vi "Process.vi"(8 "error in (no error)":errorcluster, 10 "pound in":refnum<class "Pound.lvclass">, 11 "qbus in":refnum<class "Qbus.lvclass">) -> (0 "error out":errorcluster)   [LabVIEW 2017, in "SinglePointClock.lvlib"]
doc: "This process sends data sets to the first process in the Dataflow Script for data groups that contain only single-point channels."
uses:
  <vilib>/addons/InsightCM/Devices/Shared/Common/SinglePointClock/SinglePointClock.lvlib
  <vilib>/addons/Qbus/Qbus.lvclass
  <vilib>/NI/Software Watchdog/Pound/Pound.lvclass
  <vilib>/addons/InsightCM/Devices/Shared/Common/SinglePointClock/controls/SinglePointConfig.ctl
  <vilib>/addons/TimerProcess/controls/taskType.ctl
  <vilib>/addons/InsightCM/Devices/Shared/Common/DataFlow/controls/Data.ctl
  <vilib>/addons/InsightCM/Utilities/DataAccessors/controls/wfmSGL_DVR.ctl
  <vilib>/addons/PointValueMap/controls/PointMap.ctl
  <vilib>/addons/InsightCM/Devices/Shared/Common/DataFlow/controls/Type.ctl
  <vilib>/addons/PointValueMap/subVIs/Point_Write_i32.vi
  <vilib>/addons/PointValueMap/subVIs/Point_Write_double.vi
  <vilib>/addons/TraceLogger/TraceLogger.lvlib
  <vilib>/NI/Software Watchdog/Watchdog/Watchdog.lvclass
  <vilib>/addons/InsightCM/Devices/Shared/Common/DataFlow/DataFlow.lvlib
  <vilib>/addons/PointValueMap/PointValueMap.lvlib
  <vilib>/addons/TimerProcess/TimerProcess.lvlib
  <vilib>/addons/InsightCM/Utilities/GlobalConfiguration/GlobalConfiguration.lvlib
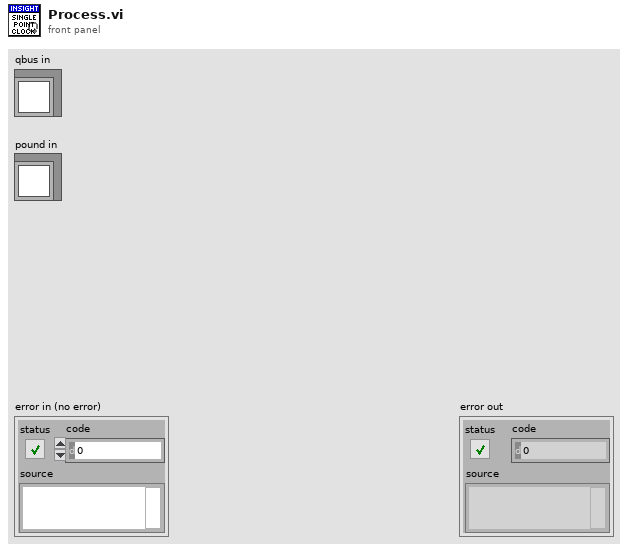
[diagram p1: front panel]
types:
  T1 = typedef "SinglePointConfig.ctl" = cluster{"AcqBlockNumber":i32, "Interval":dbl, "DataGroups":string[], "On":bool}
  T2 = typedef "TimerProcess.lvlib/taskType.ctl" = enum16{"single", "repeat"}
  T3 = typedef "DataFlow.lvlib/Type.ctl" = enum16{"High Rate", "Low Rate", "Burst Mode"}
  T4 = typedef "DataFlow.lvlib/Data.ctl" = cluster{"DataGroup":string, "Waveforms":T5, "Map":T6, "Type":T3}
  T5 = typedef "wfmSGL_DVR.ctl" = refnum<data-value>
  T6 = typedef "PointValueMap.lvlib/PointMap.ctl" = refnum<data-value>
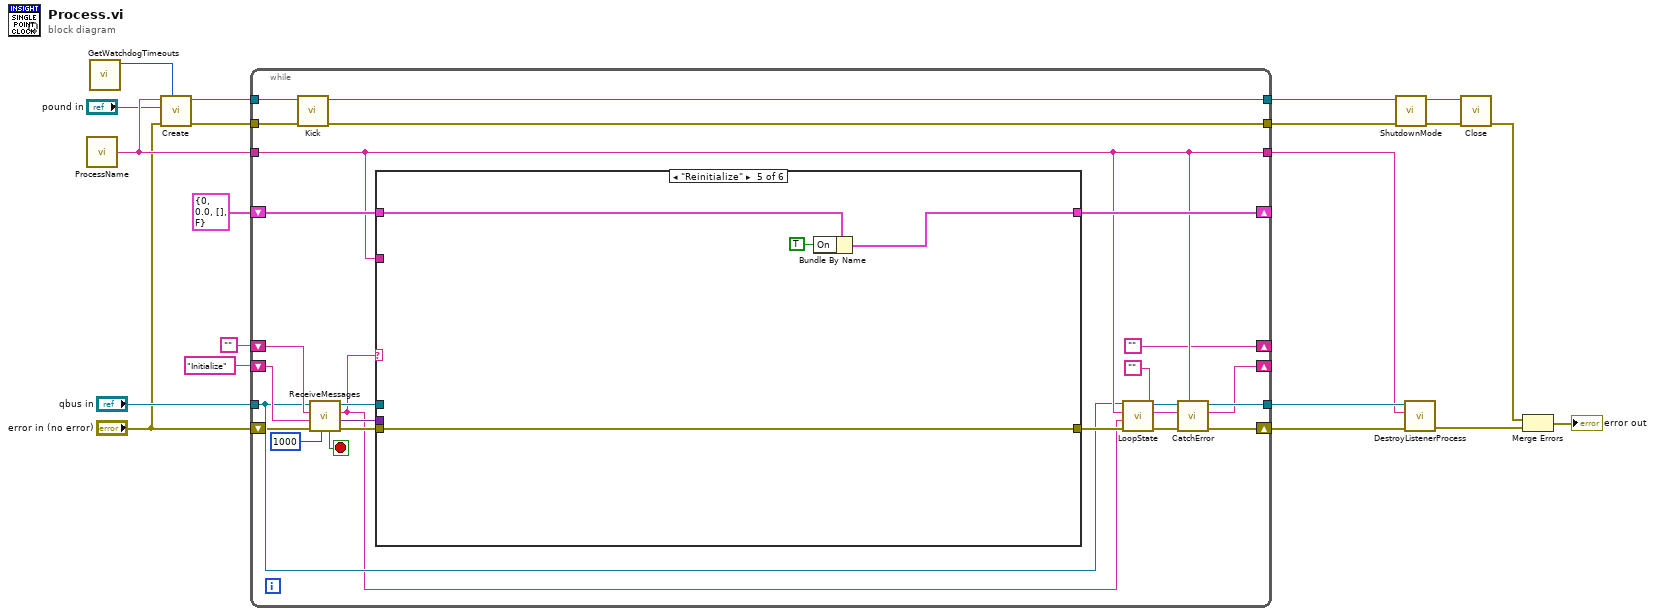
[diagram p0: block diagram]
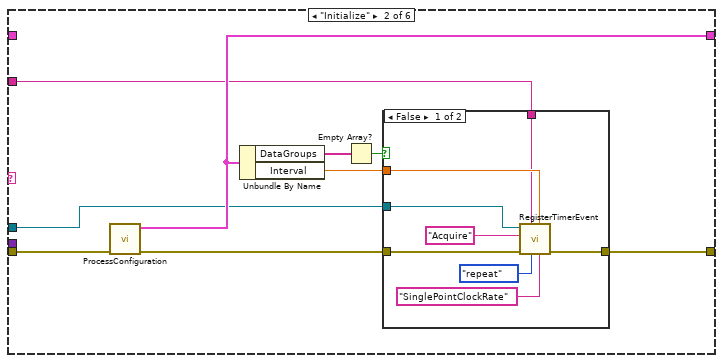
[diagram p3: hidden frame]
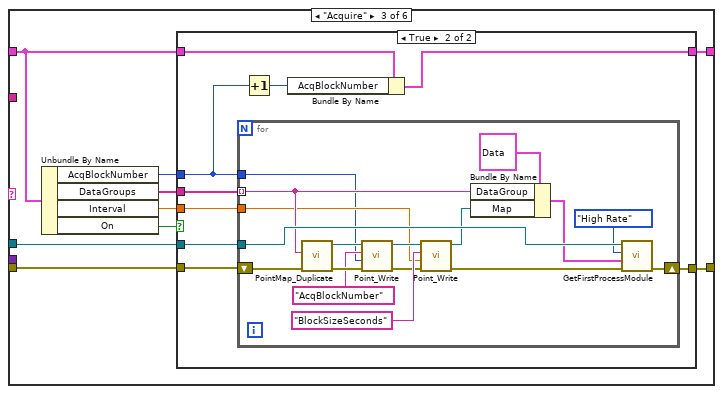
[diagram p5: hidden frame]
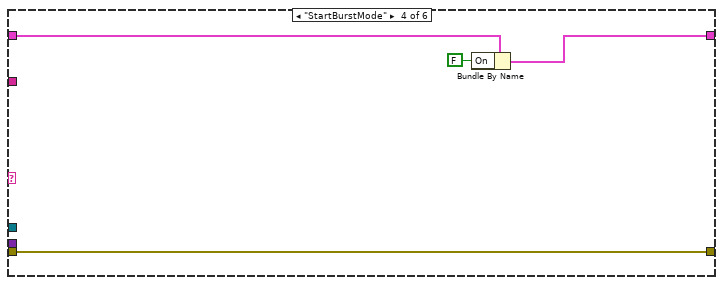
[diagram p7: hidden frame]
diagram:
  n1 = call <vilib>:"ProcessName.vi"() -> ("process name"=w15:string)  [unwired: 5 in]
  n2 = call <vilib>:"GetWatchdogTimeouts.vi"() -> ("software timeout"=w1:u32)  [unwired: 10 in, 1 out]
  n3 = call <vilib>:"Create.vi"("Execution Timeout (ms)"=w1, "error in (no error)"="error in (no error)", "Pound"="pound in", "Name"=w15) -> ("error out"=w9:errorcluster, "Watchdog"=w14:refnum<data-value>)  [unwired: 6 in]
  n4 = while {
    shift-right: [""] -> _
    shift-left: "" -> [w44]
    tunnel: "qbus in" -> [w32]
    tunnel: w15 -> [w33]
    tunnel: [w36] -> w18
    tunnel: [w33] -> w17
    shift-right: [w35] -> _
    shift-left: "Initialize" -> [w40]
    shift-right: [w38] -> _
    shift-left: T1 {"AcqBlockNumber"=0, "Interval"=0.0, "DataGroups"=[], "On"=FALSE} ("Cluster") -> [w39]
    tunnel: w14 -> [w31]
    tunnel: [w30] -> w11
    tunnel: w9 -> [w29]
    tunnel: [w27] -> w8
    shift-right: [w37] -> w19
    shift-left: "error in (no error)" -> [w28]
    stop <- w45 stop-if-true
    n5 = call <vilib>:"Kick.vi"("error in (no error)"=w29, "Watchdog"=w31) -> ("error out"=w27:errorcluster, "Watchdog"=w30:refnum<data-value>)  [unwired: 8 in]
    n6 = call <vilib>:"ReceiveMessages.vi"("timeout(100)"=1000, "error in (no error)"=w28, "priority action"=w40, "default action"=w44, "qbus in"=w32) -> ("error out"=w43:errorcluster, "msg value"=w41:variant, "action"=w26:string, "qbus out"=w42:refnum<class "Qbus.lvclass">, "exit"=w45:bool)  [unwired: 2 in]
    n7 = case shown="\"Reinitialize\"" w26 {
      tunnel: w43 -> [w47 w56 w74 w106 w110 w112]
      tunnel: w42 -> [_ w50 w73 _ _ _]
      tunnel: [w47 w54 w72 w106 w110 w112] -> w34
      tunnel: w41 -> [_ _ _ _ _ _]
      tunnel: w39 -> [w46 _ w70 w105 w109 w111]
      tunnel: [w46 w53 w69 w104 w108 w111] -> w38
      tunnel: w33 -> [_ w51 _ _ _ _]
      frame "", Default {
      }
      frame "Initialize" {
        n8 = call <vilib>:"ProcessConfiguration.vi"("error in (no error)"=w56) -> ("error out"=w55:errorcluster, "config"=w53:T1)  [unwired: 9 in]
        n9 = Unbundle By Name(w53) -> ("DataGroups"=w49:string[], "Interval"=w52:dbl)
        n10 = Empty Array?(array=w49) -> (empty?=w48:bool)
        n11 = case shown="False" w48 {
          tunnel: w55 -> [w61 w65]
          tunnel: [w60 w65] -> w54
          tunnel: w52 -> [w59 _]
          tunnel: w51 -> [w58 _]
          tunnel: w50 -> [w57 _]
          frame False {
            n12 = call <vilib>:"RegisterTimerEvent.vi"("timer task name"="SinglePointClockRate" ("Name"), "interval (sec)"=w59, "type"=taskType."repeat", "process name"=w58, "error in (no error)"=w61, "callback action"="Acquire", "qbus in"=w57) -> ("error out"=w60:errorcluster)  [unwired: 3 in, 1 out]
          }
          frame True {
          }
        }
      }
      frame "Acquire" {
        n13 = Unbundle By Name(w70) -> ("AcqBlockNumber"=w67:i32, "DataGroups"=w71:string[], "Interval"=w68:dbl, "On"=w66:bool)
        n14 = case shown="True" w66 {
          tunnel: w74 -> [w75 w85]
          tunnel: w73 -> [_ w84]
          tunnel: [w75 w83] -> w72
          tunnel: w71 -> [_ w82]
          tunnel: w70 -> [w76 w80]
          tunnel: [w76 w79] -> w69
          tunnel: w68 -> [_ w78]
          tunnel: w67 -> [_ w77]
          frame False {
          }
          frame True {
            n15 = for {
              tunnel: w84 -> [w102]
              shift-right: [w101] -> w83
              shift-left: w85 -> [w96]
              tunnel: w82 -> [w89] mode=indexing
              tunnel: w78 -> [w88]
              tunnel: w77 -> [w87]
              n16 = call <vilib>:"PointMap_Duplicate.vi"("error in (no error)"=w96, "Source Map Name"=w89) -> ("error out"=w91:errorcluster, "Map Out"=w94:T6)  [unwired: 8 in]
              n17 = call-poly <vilib>:"Point_Write.vi"("Error In"=w91, "Value"=w87, "Tag"="AcqBlockNumber", "Map"=w94) -> ("Error Out"=w92:errorcluster, "Map Out"=w93:T6)  [unwired: 6 in]
              n18 = call-poly <vilib>:"Point_Write.vi"("Error In"=w92, "Value"=w88, "Tag"="BlockSizeSeconds", "Map"=w93) -> ("Error Out"=w99:errorcluster, "Map Out"=w98:T6)  [unwired: 6 in]
              n19 = Bundle By Name(cluster=T4 {"DataGroup"="", "Waveforms"=refnum, "Map"=refnum, "Type"=enum."High Rate"} ("data"), "DataGroup"=w89, "Map"=w98) -> (w100:T4)
              n20 = call <vilib>:"GetFirstProcessModule.vi"("error in (no error)"=w99, "data"=w100, "type"=Type."High Rate", "Qbus in"=w102) -> ("error out"=w101:errorcluster)  [unwired: 6 in, 1 out]
            }
            n21 = Increment(x=w77) -> (x+1=w81:i32)
            n22 = Bundle By Name(cluster=w80, "AcqBlockNumber"=w81) -> (w79:T1)
          }
        }
      }
      frame "StartBurstMode" {
        n23 = Bundle By Name(cluster=w105, "On"=FALSE) -> (w104:T1)
      }
      frame "Reinitialize" {
        n24 = Bundle By Name(cluster=w109, "On"=TRUE) -> (w108:T1)
      }
      frame "Exit" {
      }
    }
    n25 = call <vilib>:"LoopState.vi"("error in (no error)"=w34, "loop action"=w26, "process name"=w33, "Qbus in"=w32) -> ("error out"=w21:errorcluster, "Qbus out"=w22:refnum<class "Qbus.lvclass">)  [unwired: 6 in]
    n26 = call <vilib>:"CatchError.vi"("source"=w33, "error in (no error)"=w21, "next action in"="", "Qbus in"=w22) -> ("error out"=w37:errorcluster, "next action out"=w35:string, "Qbus out"=w36:refnum<class "Qbus.lvclass">)  [unwired: 5 in]
  }
  n27 = call <vilib>:"ShutdownMode.vi"("error in (no error)"=w8, "Watchdog"=w11) -> ("error out"=w10:errorcluster, "Watchdog"=w12:refnum<data-value>)  [unwired: 8 in]
  n28 = call <vilib>:"DestroyListenerProcess.vi"("error in (no error)"=w19, "process name"=w17, "Qbus in"=w18) -> ("error in (no error)"=w7:errorcluster)  [unwired: 7 in, 1 out]
  n29 = call <vilib>:"Close.vi"("error in (no error)"=w10, "Watchdog"=w12) -> ("error out"=w6:errorcluster)  [unwired: 9 in]
  n30 = Merge Errors(w6, w7) -> (→"error out":errorcluster)
